vi "Image_Snap_Enqueue_2.0.vi"(0 "Data":T1={"Camera 1"={"Camera1"="", "Cam 1"=FALSE, "CAM1 Model"=enum."a2A5328-15ucBAS", "Cam1 ID"=0}, "Camera 2"={"Camera2"="", "Cam 2"=FALSE, "CAM2 Model"=enum."a2A5328-15ucBAS", "Cam2 ID"=0}, "Image"={"Camera1_Img"=refnum, "Camera2_Img"=refnum, "Img1_Orig_Disp"=refnum, "Img2_Orig_Disp"=refnum, "Img1_Orig_RGB"=refnum, "Img2_Orig_RGB"=refnum, "Blue_Plane_Extract"=refnum, "Subtracted_Plane"=refnum, "Img1_Binary"=refnum, "Img2_Binary"=refnum, "Crop_Mask"=refnum, "Img1_Save"=refnum, "Img2_Save"=refnum, "Img1_Cali_Full"=refnum, "Img2_Cali_Full"=refnum, "Img1_Cali_Detect"=refnum, "Img2_Cali_Detect"=refnum}, "Ques"={"Cam 1 queue"=refnum, "Cam 2 queue"=refnum, "Cam 1 - save queue"=refnum, "Cam 2 - save queue"=refnum, "Image Process Queue Size"=500, "Image Save Queue Size"=500, "Overload threshold"=500, "Max large object threshold"=0}, "Arduino SRS"={"Pinch-valve"="", "Actuator"=FALSE, "Open(T)/Close(F)"=FALSE, "Arduino Uno"=""}, "Pump"={"Port"="", "Connection"=FALSE, "Pump State"=FALSE, "Pump Model"=enum."XLP6000", "Pump size"=FALSE, "Flush Size"=0, "Dispense Speed"=100, "Command"="", "Pump"=""}, "Camera settings"={"Detection settings"={"Sample size threshold"=500, "Detection Region %"=30.0, "Timeout Sample"=200}, "Lens/camera settings"={"Aperture"=enum."Item 0", "Legacy Cam Attributes"=FALSE, "Max Framerate"=100, "Exposure Time"=1000.0, "Framerate"=15}, "Crop settings"={"Cam1"={"Rectangle 1"={"Left"=0, "Top"=0, "Right"=0, "Bottom"=0, "Rotation"=0.0}, "Camera Orientation 1"="", "Pixel to mm 1"=0.0}, "Cam2"={"Rectangle 2"={"Left"=0, "Top"=0, "Right"=0, "Bottom"=0, "Rotation"=0.0}, "Camera Orientation 2"="", "Pixel to mm 2"=0.0}}}, "Arduino ISS"={"Mega F3"="", "Phase3"=FALSE, "Barcode"="", "Sorting sys."=FALSE, "Initial size"=0.0, "Size Interval"=0.0, "Mun. of containers"=0.0, "Container nr."=0.0, "Arduino Mega"=""}, "Img_Capt"=FALSE, "Empty_Refill"=FALSE, "I don't think is in use"={"Crop"=FALSE, "Light intensity"=100, "Empty start"=1}, "Img_Capt Begin"=FALSE, "Extended setup"={"Location"="Station", "Latitude"="Station", "Longitude"="Station", "Determiner"="Station", "Sex"="Station", "Station"="", "Collection date"=""}, "Main interface"={"Sample Name"="Test Sample", "Operator"="JFR", "Species Name"="", "Other Notes"=""}, "Tap1"=0, "SystemVersion"=0, "System Serial"="", "Flush Insect"=FALSE, "Exit"=FALSE, "Kuvette Full"=FALSE, "Core JKI"={"Current VI Reference"=refnum, "Close Panel on Exit?"=FALSE}, "Calibration"={"Calibration 1"=path "C:/Users/au540322/Desktop/IHS_Project/images/Debris/Debris_0/Debris_0_2019_06_01-23-32-49-686.PNG", "Calibration 2"=path "C:/Users/au540322/Desktop/IHS_Project/images/Debris/Debris_0/Debris_0_2019_06_01-23-32-49-686.PNG", "Detect 1"=path "C:/Users/au540322/Desktop/IHS_Project/images/Debris/Debris_0/Debris_0_2019_06_01-23-32-49-686.PNG", "Detect 2"=path "C:/Users/au540322/Desktop/IHS_Project/images/Debris/Debris_0/Debris_0_2019_06_01-23-32-49-686.PNG"}} {"SystemVersion" items=["Standard", "XL"]; "Tap1" items=["Session Data", "Extended Setup", "Buffer", "Camera", "Dispenser", "Stats", "Connections"]; "I don't think is in use"."Empty start" min=1; "I don't think is in use"."Light intensity" scale=0.0..100.0; "Camera settings"."Crop settings"."Cam2"."Rectangle 2"."Rotation" format="%.2f"; "Camera settings"."Crop settings"."Cam2"."Rectangle 2"."Left" scale=0.0..1024.0; "Camera settings"."Crop settings"."Cam2"."Rectangle 2"."Right" scale=0.0..1024.0; "Camera settings"."Crop settings"."Cam1"."Rectangle 1"."Rotation" format="%.2f"; "Camera settings"."Crop settings"."Cam1"."Rectangle 1"."Left" scale=0.0..1024.0; "Camera settings"."Crop settings"."Cam1"."Rectangle 1"."Right" scale=0.0..1024.0; "Camera settings"."Lens/camera settings"."Framerate" min=1; "Camera settings"."Lens/camera settings"."Max Framerate" min=1; "Camera settings"."Detection settings"."Sample size threshold" min=1; "Pump"."Dispense Speed" min=1; "Pump"."Flush Size" min=0 max=6000 step=100; "Ques"."Overload threshold" min=1; "Ques"."Image Save Queue Size" min=1; "Ques"."Image Process Queue Size" min=1}, 5 "Camera queue":refnum<queue>, 7 "Camera":T5, 9 "Detect Movement":bool, 11 "error in":errorcluster) -> (4 "Image out":T3, 15 "error out":errorcluster)   [LabVIEW 2024]
doc: "Takes picture from single camera and converts to array output."
uses:
  <vilib>/vision/Image Controls.llb/IMAQ Image.ctl
  Camera_ID.ctl
  controls/Data_JKI.ctl
  <vilib>/userDefined/High Color/IMAQdx.ctl
  <vilib>/vision/driver/NI_Vision_Acquisition_Software.lvlib
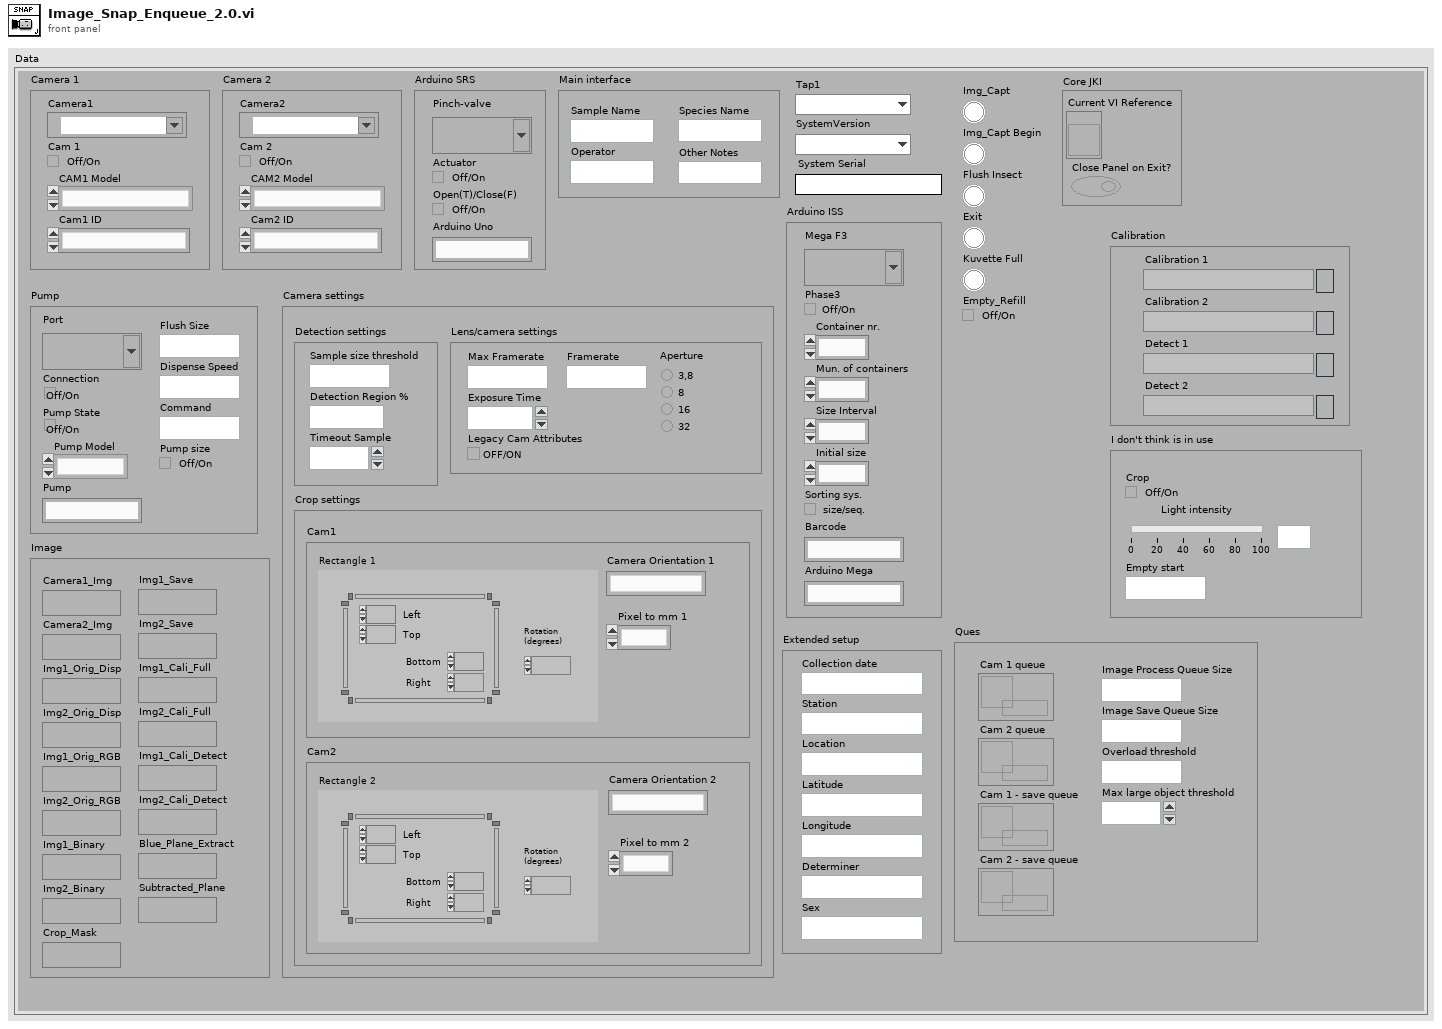
[diagram p1: front panel]
types:
  T1 = typedef "Data_JKI.ctl" = cluster{"Camera 1":cluster{"Camera1":T2, "Cam 1":bool, "CAM1 Model":enum16{"a2A5328-15ucBAS", "acA1920-155uc"}, "Cam1 ID":i32}, "Camera 2":cluster{"Camera2":T2, "Cam 2":bool, "CAM2 Model":enum16{"a2A5328-15ucBAS", "acA1920-155uc"}, "Cam2 ID":i32}, "Image":cluster{"Camera1_Img":T3, "Camera2_Img":T3, "Img1_Orig_Disp":T3, "Img2_Orig_Disp":T3, "Img1_Orig_RGB":T3, "Img2_Orig_RGB":T3, "Blue_Plane_Extract":T3, "Subtracted_Plane":T3, "Img1_Binary":T3, "Img2_Binary":T3, "Crop_Mask":T3, "Img1_Save":T3, "Img2_Save":T3, "Img1_Cali_Full":T3, "Img2_Cali_Full":T3, "Img1_Cali_Detect":T3, "Img2_Cali_Detect":T3}, "Ques":cluster{"Cam 1 queue":refnum<queue>, "Cam 2 queue":refnum<queue>, "Cam 1 - save queue":refnum<queue>, "Cam 2 - save queue":refnum<queue>, "Image Process Queue Size":i32, "Image Save Queue Size":i32, "Overload threshold":i32, "Max large object threshold":i32}, "Arduino SRS":cluster{"Pinch-valve":refnum<visa-resource-name>, "Actuator":bool, "Open(T)/Close(F)":bool, "Arduino Uno":string}, "Pump":cluster{"Port":refnum<visa-resource-name>, "Connection":bool, "Pump State":bool, "Pump Model":enum16{"XLP6000", "XL1000"}, "Pump size":bool, "Flush Size":i32, "Dispense Speed":i32, "Command":string, "Pump":string}, "Camera settings":cluster{"Detection settings":cluster{"Sample size threshold":i32, "Detection Region %":dbl, "Timeout Sample":i32}, "Lens/camera settings":cluster{"Aperture":enum32{"Item 0", "Item 1", "Item 2", "Item 3"}, "Legacy Cam Attributes":bool, "Max Framerate":i32, "Exposure Time":dbl, "Framerate":i32}, "Crop settings":cluster{"Cam1":cluster{"Rectangle 1":T4, "Camera Orientation 1":string, "Pixel to mm 1":dbl}, "Cam2":cluster{"Rectangle 2":T4, "Camera Orientation 2":string, "Pixel to mm 2":dbl}}}, "Arduino ISS":cluster{"Mega F3":refnum<visa-resource-name>, "Phase3":bool, "Barcode":string, "Sorting sys.":bool, "Initial size":dbl, "Size Interval":dbl, "Mun. of containers":dbl, "Container nr.":dbl, "Arduino Mega":string}, "Img_Capt":bool, "Empty_Refill":bool, "I don't think is in use":cluster{"Crop":bool, "Light intensity":i32, "Empty start":u32}, "Img_Capt Begin":bool, "Extended setup":cluster{"Location":string, "Latitude":string, "Longitude":string, "Determiner":string, "Sex":string, "Station":string, "Collection date":string}, "Main interface":cluster{"Sample Name":string, "Operator":string, "Species Name":string, "Other Notes":string}, "Tap1":u16, "SystemVersion":u16, "System Serial":string, "Flush Insect":bool, "Exit":bool, "Kuvette Full":bool, "Core JKI":cluster{"Current VI Reference":refnum<vi>, "Close Panel on Exit?":bool}, "Calibration":cluster{"Calibration 1":path, "Calibration 2":path, "Detect 1":path, "Detect 2":path}}
  T2 = typedef "IMAQdx.ctl" = refnum<k21>
  T3 = typedef "IMAQ Image.ctl" = refnum<image>
  T4 = typedef "IMAQ Rectangle" = cluster{"Left":i32, "Top":i32, "Right":i32, "Bottom":i32, "Rotation":dbl}
  T5 = typedef "Camera_ID.ctl" = enum16{"Camera 1", "Camera 2"}
  T6 = cluster{"Image Pixels (U32)":u32[][], "Detect Movement":bool, "date/time string":string}
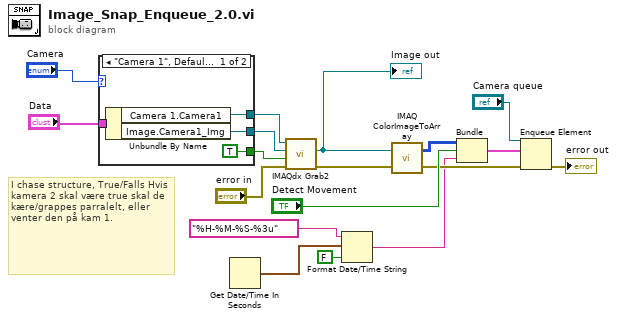
[diagram p0: block diagram]
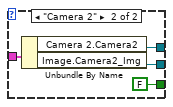
[diagram p2: hidden frame]
diagram:
  # "I chase structure, True/Falls Hvis kamera 2 skal være true skal de kære/grappes parralelt, eller venter den på kam 1."
  n1 = case shown="\"Camera 1\", Default" "Camera" {
    tunnel: "Data" -> [w20 w26]
    tunnel: [w22 w25] -> w13
    tunnel: [w21 w24] -> w18
    tunnel: [TRUE ("Wait for Next Buffer? (Yes)") FALSE ("Wait for Next Buffer? (Yes)")] -> w14
    frame "Camera 1", Default {
      n2 = Unbundle By Name(w20) -> ("Camera 1.Camera1"=w22:T2, "Image.Camera1_Img"=w21:T3)
    }
    frame "Camera 2" {
      n3 = Unbundle By Name(w26) -> ("Camera 2.Camera2"=w25:T2, "Image.Camera2_Img"=w24:T3)
    }
  }
  n4 = Get Date/Time In Seconds() -> (seconds since 1Jan1904=w2:timestamp)
  n5 = call <vilib>:"IMAQdx Grab2.vi"("error in"="error in", "Wait for Next Buffer? (Yes)"=w14, "Image In"=w18, "Session In"=w13) -> ("error out"=w9:errorcluster, "Image Out"=w10:T3)  [unwired: 4 in, 2 out]
  "Image out" <- w10
  n6 = Format Date/Time String(time format string (%c)="%H-%M-%S-%3u", seconds (now)=w2, UTC format=FALSE) -> (date/time string=w4:string)
  n7 = call "IMAQ ColorImageToArray"("Image"=w10, "error in (no error)"=w9) -> ("Image Pixels (U32)"=w8:u32[][], "error out"=w11:errorcluster)  [unwired: 2 in, 1 out]
  n8 = Bundle("Image Pixels (U32)"=w8, "Detect Movement"="Detect Movement", "date/time string"=w4) -> (w3:T6)  [unwired: 1 in]
  n9 = Enqueue Element(queue="Camera queue", element=w3, error in (no error)=w11) -> (error out=→"error out":errorcluster)  [unwired: 1 in, 2 out]
